vi "Load Offsets.vi"(8 "error in (no error)":errorcluster) -> (0 "error out":errorcluster)   [LabVIEW 2009]
uses:
  lib/Apps/App Parameters Actions.ctl
  lib/Logging/LogFileType.ctl
  lib/Data Access Objects/Metadata/LBCB Number.ctl
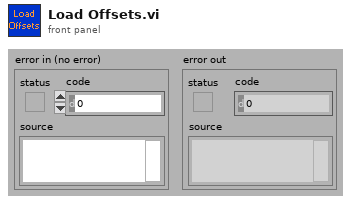
[diagram p1: front panel]
types:
  T1 = typedef "LogFileType.ctl" = enum16{"Continuous", "Step", "Volts", "Offsets", "Mixed Mode State", "DLL  Errors", "End List"}
  T2 = typedef "App Parameters Actions.ctl" = enum16{"Init", "Get", "Set"}
  T3 = typedef "App Parameters.ctl" = cluster{"Monitor Loop":T4, "Ramp Time":T4, "Log Loop":T4, "TCP to DAQ":T4, "Logging Directory":path, "Log File Size (MBytes)":i64, "Volt Logging Loop":T4}
  T4 = typedef "Timing Parameters.ctl" = cluster{"Interval":dbl, "Rate ":dbl}
  T5 = typedef "LBCB Number.ctl" = enum16{"LBCB1", "LBCB2"}
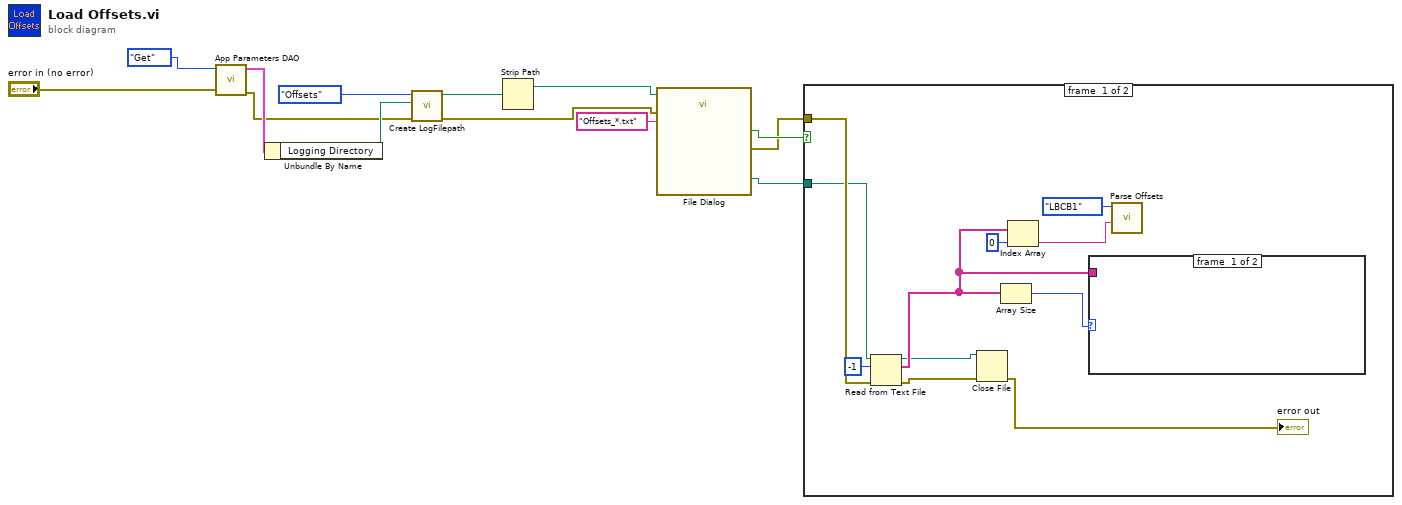
[diagram p0: block diagram]
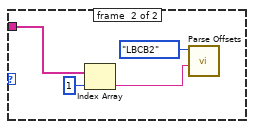
[diagram p2: hidden frame]
diagram:
  n1 = call "App Parameters DAO.vi"("error in (no error)"="error in (no error)", "Actions"=App_Parameters_Actions."Get" ("App Parameter Actions")) -> ("error out"=w10:errorcluster, "Application Timing and Logging Out"=w13:T3)  [unwired: 2 in, 6 out]
  n2 = Unbundle By Name(w13) -> ("Logging Directory"=w12:path)
  n3 = call "Create LogFilepath.vi"("error in (no error)"=w10, "Log Directory"=w12, "LogFile Type"=LogFileType."Offsets") -> ("error out"=w2:errorcluster, "Logfile Path"=w7:path)  [unwired: 7 out]
  n4 = Strip Path(path=w7) -> (stripped path=w5:path)  [unwired: 1 out]
  n5 = call "File Dialog"("start path"=w5, "error in"=w2, "pattern (all files)"="Offsets_*.txt") -> ("selected path"=w6:path, "cancelled"=w3:bool, "error out"=w1:errorcluster)  [unwired: 9 in, 1 out]
  n6 = case shown="False" w3 {
    tunnel: w1 -> [w24 _]
    tunnel: w6 -> [w23 _]
    frame #0 {
      n7 = Read from Text File(file (use dialog)=w23, count=-1, error in=w24) -> (refnum out=w16:refnum<file>, text=w17:string[], error out=w15:errorcluster)  [unwired: 1 in, 1 out]
      n8 = Close File(refnum=w16, error in=w15) -> (error out=→"error out":errorcluster)  [unwired: 1 out]
      n9 = Array Size(array=w17) -> (size(s)=w21:i32)
      n10 = Index Array(array=w17, index=0) -> (element=w19:string)
      n11 = case shown="2" w21 {
        tunnel: w17 -> [_ w25]
        frame #0 {
        }
        frame #1 {
          n12 = Index Array(array=w25, index=1) -> (element=w27:string)
          n13 = call "Parse Offsets.vi"("Line"=w27, "LBCB Selected"=LBCB_Number."LBCB2") -> ()  [unwired: 10 in]
        }
      }
      n14 = call "Parse Offsets.vi"("Line"=w19, "LBCB Selected"=LBCB_Number."LBCB1") -> ()  [unwired: 10 in]
    }
    frame #1 {
    }
  }
